vi "Calculate position.vi"(5 "Fs reading":dbl, 6 "Gyro LSB":dbl, 7 "Gyro %":dbl, 8 "Acc position (radians)":dbl, 9 "Gyro position (LSB)":i16, 11 "Old position":dbl) -> (3 "New position":dbl)   [LabVIEW 2017]
uses:
  <userlib>/_MGI/Numeric/Coercion/MGI Radians to Degrees/MGI Radians to Degrees DBL.vi
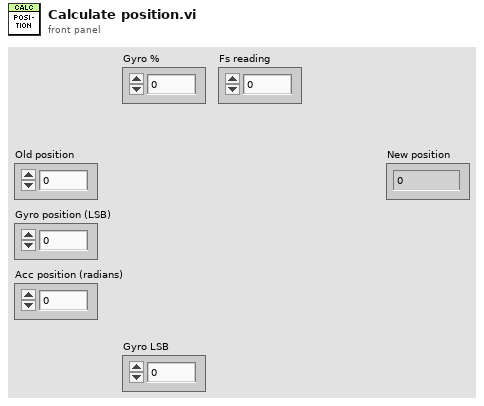
[diagram p1: front panel]
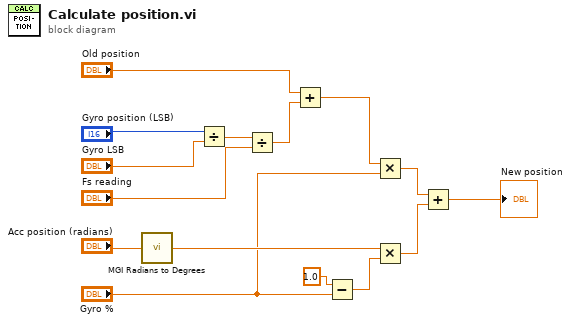
[diagram p0: block diagram]
diagram:
  n1 = call-poly <userlib>:"MGI Radians to Degrees.vi"("Radians"="Acc position (radians)") -> ("Degrees"=w13:dbl)
  n2 = Divide(x="Gyro position (LSB)", y="Gyro LSB") -> (x/y=w9:dbl)
  n3 = Divide(x=w9, y="Fs reading") -> (x/y=w8:dbl)
  n4 = Add(x="Old position", y=w8) -> (x+y=w6:dbl)
  n5 = Subtract(x=1.0, y="Gyro %") -> (x-y=w10:dbl)
  n6 = Multiply(x=w6, y="Gyro %") -> (x*y=w4:dbl)
  n7 = Multiply(x=w13, y=w10) -> (x*y=w5:dbl)
  n8 = Add(x=w4, y=w5) -> (x+y=→"New position":dbl)
